vi "Get Path.vi"(8 "error in (no error)":errorcluster, 11 "Cookie in":refnum<class "Cookie.lvclass">) -> (0 "error out":errorcluster, 2 "Cookie Path":string, 3 "Cookie out":refnum<class "Cookie.lvclass">)   [LabVIEW 2020, in "HTTP Utils.lvlib" / "Cookie.lvclass"]
uses:
  Cookie.lvclass
  Cookie.lvclass/Cookie.ctl
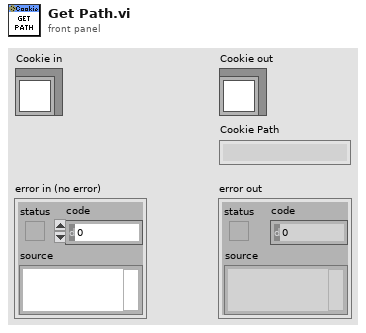
[diagram p1: front panel]
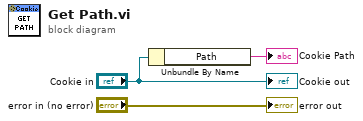
[diagram p0: block diagram]
diagram:
  n1 = Unbundle By Name("Cookie in") -> ("Path"=→"Cookie Path":string)
  "error out" <- "error in (no error)"
  "Cookie out" <- "Cookie in"
